vi "CD Init Outgoing Cyclic Signals.vi"(6 "Memory Table Offset":u32, 8 "error in":errorcluster, 9 "database":T1, 10 "can port":string, 11 "XNET Cluster":refnum<k21>) -> (0 "error out":errorcluster, 1 "Outgoing Cyclic Configuraiton":T5 {"Outgoing Cyclic Frame"."Transmit Propreties"."Transmit Time" format="%#_p"}, 2 "initial values":dbl[](array[numeric]), 3 "channels":refnum<class "TBM channel.lvclass">[](array[class]), 5 "outputs":T4[](array[typedef]), 7 "output IDs":string[](array[string]))   [LabVIEW 2013, in "J1939.lvlib"]
uses:
  J1939.lvlib
  CD Outgoing Cyclic Configuration.ctl
  CD Outgoing Cyclic Frame Pairs.ctl
  API Types/XNET Frame Event Properties.ctl
  module/configuration/Signal Mapping.ctl
  <vilib>/NI/Tag Bus/tag/Data Type.ctl
  <vilib>/NI/Tag Bus Module Framework/channel/TBM channel.lvclass
  CD Conversion Lookup Table Parameters Cluster.ctl
  Configuration/TypeDefs/J1939 db.ctl
  Configuration/TypeDefs/J1939 db frame.ctl
  Configuration/TypeDefs/J1939 db signal.ctl
  Configuration/TypeDefs/J1939 db frame direction.ctl
  <vilib>/NI/Tag Bus Module Framework/channel/channel classification.ctl
  <vilib>/NI/Tag Bus/tag/tag descriptor.lvclass/tag descriptor.ctl
  Frame Conversion/Common Conversions.vi
  Frame Conversion/Convert CAN Arb ID to J1939 ID.vi
  <vilib>/xnet/xnet.llb/XNET Create Session (Conversion).vi
  <resource>/objmgr/xnet.rc
  <vilib>/NI/Tag Bus/tag/tag descriptor.lvclass
  module/configuration/J1939 configuration.lvclass
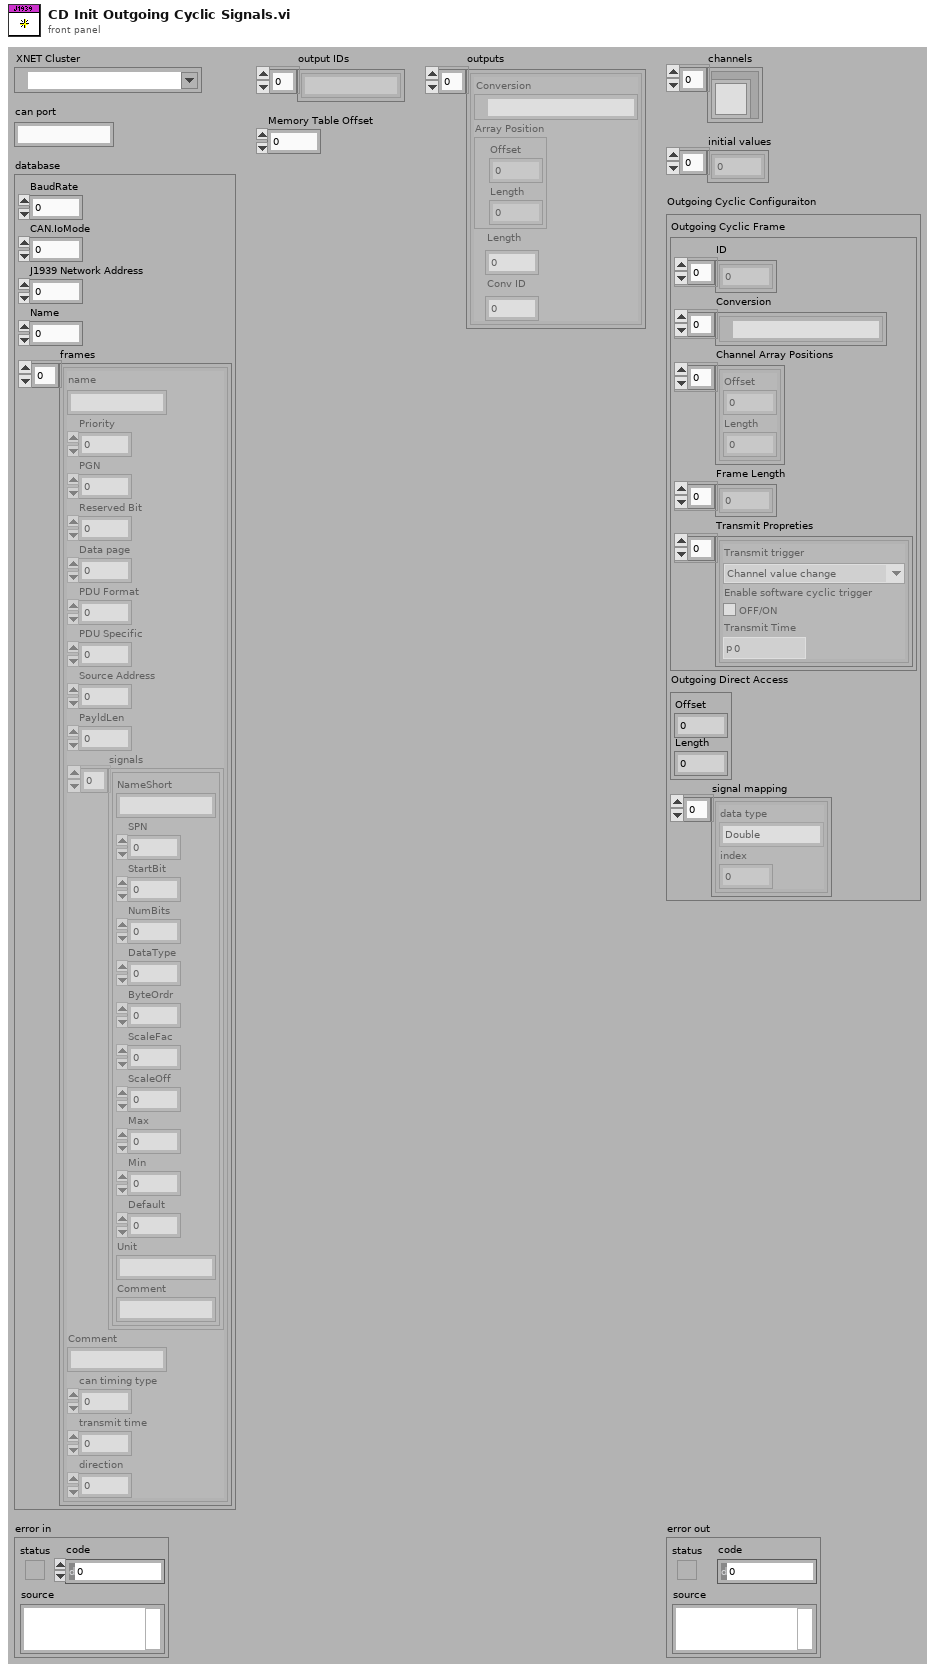
[diagram p1: front panel]
types:
  T1 = typedef "J1939.lvlib/J1939 db.ctl" = cluster{"BaudRate":u32, "CAN.IoMode":u32, "J1939 Network Address":u8, "Name":u64, "frames":T2[]}
  T2 = typedef "J1939.lvlib/J1939 db frame.ctl" = cluster{"name":string, "Priority":u8, "PGN":u32, "Reserved Bit":u8, "Data page":u8, "PDU Format":u8, "PDU Specific":u8, "Source Address":u8, "PayldLen":u32, "signals":T3[], "Comment":string, "can timing type":u32, "transmit time":dbl, "direction":u16}
  T3 = typedef "J1939.lvlib/J1939 db signal.ctl" = cluster{"NameShort":string, "SPN":i32, "StartBit":u32, "NumBits":u32, "DataType":u32, "ByteOrdr":u32, "ScaleFac":dbl, "ScaleOff":dbl, "Max":dbl, "Min":dbl, "Default":dbl, "Unit":string, "Comment":string}
  T4 = typedef "J1939.lvlib/CD Conversion Lookup Table Parameters Cluster.ctl" = cluster{"Conversion":refnum<k21>, "Array Position":cluster{"Offset":u32, "Length":u32}, "Length":u32, "Conv ID":u32}
  T5 = typedef "J1939.lvlib/CD Outgoing Cyclic Configuration.ctl" = cluster{"Outgoing Cyclic Frame":T6, "Outgoing Direct Access":cluster{"Offset":u32, "Length":u32}, "signal mapping":T8[]}
  T6 = typedef "J1939.lvlib/CD Outgoing Cyclic Frame Pairs.ctl" = cluster{"ID":u32[], "Conversion":refnum<k21>[], "Channel Array Positions":cluster{"Offset":u32, "Length":u32}[], "Frame Length":u32[], "Transmit Propreties":T7[]}
  T7 = typedef "J1939.lvlib/XNET Frame Event Properties.ctl" = cluster{"Transmit trigger":enum16{"Channel value change"}, "Enable software cyclic trigger":bool, "Transmit Time":dbl}
  T8 = typedef "J1939 configuration.lvclass/Signal Mapping.ctl" = cluster{"data type":T9, "index":i32}
  T9 = typedef "tag bus.lvlib/tag descriptor.lvclass/Data Type.ctl" = enum16{"Double", "Single", "I64", "I32", "I16", "I8", "U64", "U32", "U16", "U8", "Boolean", "String", "Array of Double", "Array of Single", "Array of I64", "Array of I32", "Array of I16", "Array of I8", "Array of U64", "Array of U32", "Array of U16", "Array of U8", "Array of Boolean", "Array of String"}
  T10 = typedef "J1939.lvlib/J1939 db frame direction.ctl" = enum16{"Input", "Output", "Input+Output"}
  T11 = typedef "TBM channel.lvclass/channel classification.ctl" = enum16{"input data", "output data", "processing parameter", "processing result"}
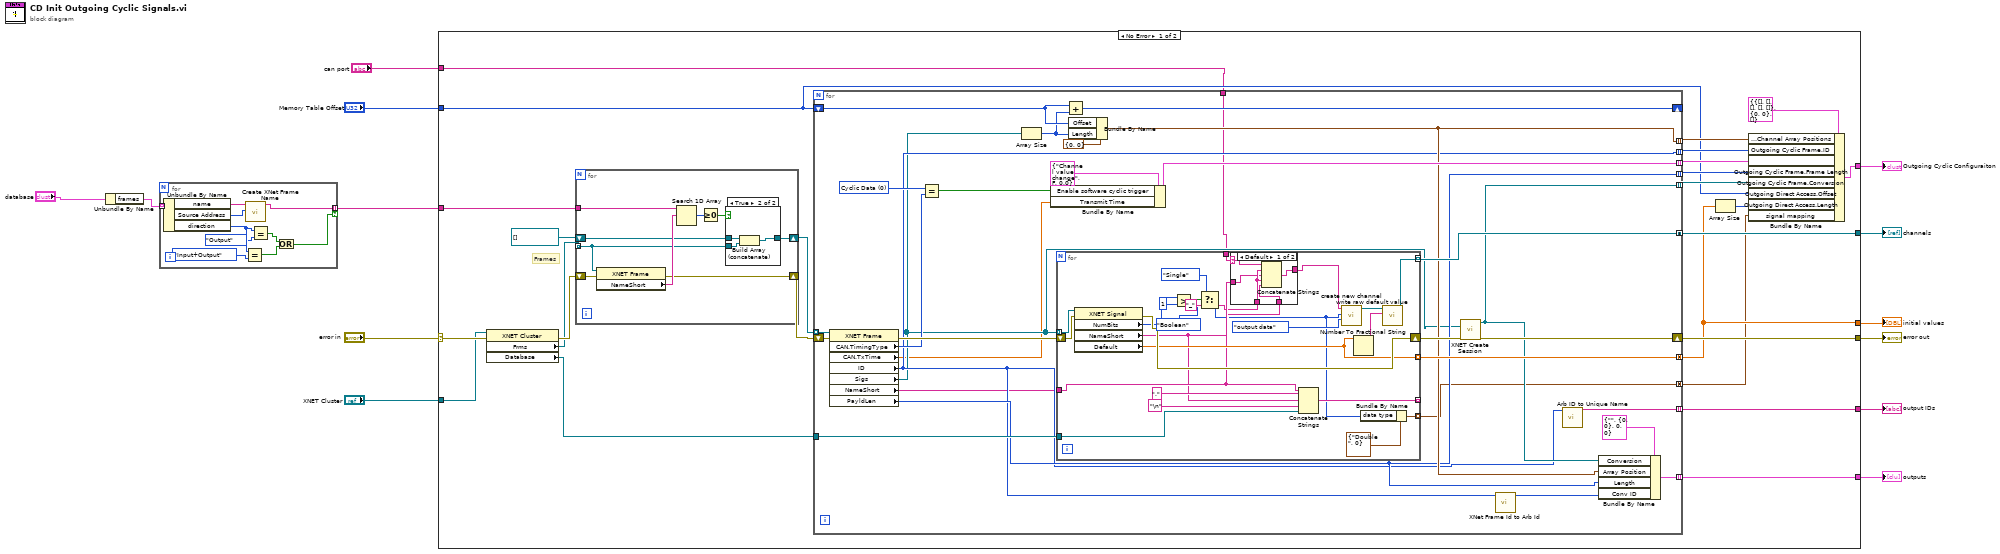
[diagram p0: block diagram]
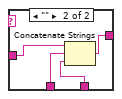
[diagram p3: hidden frame]
diagram:
  n1 = Unbundle By Name("database") -> ("frames"=w3:T2[])
  n2 = for {
    tunnel: w3 -> [w23] mode=indexing
    tunnel: [w20] -> w1 mode=indexing if=w14
    n3 = Unbundle By Name(w23) -> ("name"=w22:string, "Source Address"=w21:u8, "direction"=w19:u16)
    n4 = Equal?(x=w19, y=J1939_db_frame_direction."Input+Output" ("Direction")) -> (x = y?=w16:bool)
    n5 = call "Create XNet Frame Name.vi"("Source Address"=w21, "name"=w22) -> ("String"=w20:string)  [unwired: 8 in, 1 out]
    n6 = Equal?(x=w19, y=J1939_db_frame_direction."Output" ("Direction")) -> (x = y?=w15:bool)
    n7 = Or(x=w15, y=w16) -> (x .or. y?=w14:bool)
  }
  n8 = case shown="No Error" "error in" {
    selector: "error in" -> [w41 w126]
    tunnel: [w48 _] -> w11
    tunnel: [w39 w126] -> w13
    tunnel: "Memory Table Offset" -> [w30 _]
    tunnel: "XNET Cluster" -> [w40 _]
    tunnel: [w33 _] -> w9
    tunnel: [w32 _] -> w8
    tunnel: [w31 _] -> w7
    tunnel: [w29 _] -> w6
    tunnel: "can port" -> [w25 _]
    tunnel: w1 -> [w24 _]
    frame No Error {
      # "Frames"
      n9 = property class="XNET Cluster"(reference=w40, error in=w41) -> (error out=w38:errorcluster, "Frms"=w37:refnum<k21>[], "Database"=w26:refnum<k21>)  [unwired: 1 out]
      n10 = for {
        tunnel: w37 -> [w53] mode=indexing
        tunnel: w24 -> [w57]
        shift-right: [w52] -> w35
        shift-left: refnum<k21>[] [] -> [w49]
        shift-right: [w50] -> w34
        shift-left: w38 -> [w51]
        n11 = property class="XNET Frame"(reference=w53, error in=w51) -> (error out=w50:errorcluster, "NameShort"=w56:string)  [unwired: 1 out]
        n12 = Search 1D Array(1D array=w57, element=w56) -> (index of element=w55:i32)  [unwired: 1 in]
        n13 = Greater Or Equal To 0?(x=w55) -> (x >= 0?=w54:bool)
        n14 = case shown="True" w54 {
          tunnel: w49 -> [w58 w61]
          tunnel: w53 -> [_ w60]
          tunnel: [w58 w59] -> w52
          frame False {
          }
          frame True {
            n15 = Build Array (concatenate)(w61, w60) -> (w59:refnum<k21>[])
          }
        }
      }
      n16 = for {
        tunnel: [w73] -> w47 mode=indexing
        tunnel: [w69] -> w42 mode=indexing
        shift-right: [w91] -> _
        shift-left: w30 -> [w89]
        tunnel: [w72] -> w46 mode=indexing
        tunnel: [w71] -> w45 mode=indexing
        tunnel: [w79] -> w44 mode=indexing
        tunnel: w35 -> [w87] mode=indexing
        shift-right: [w82] -> w39
        shift-left: w34 -> [w86]
        tunnel: w26 -> [w81]
        tunnel: [w77] -> w33 mode=concatenating
        tunnel: [w76] -> w29 mode=concatenating
        tunnel: [w68] -> w32 mode=indexing
        tunnel: [w74] -> w31 mode=indexing
        tunnel: [w67] -> w27 mode=concatenating
        tunnel: w25 -> [w64]
        w83 = u32 0 items=["Cyclic Data", "Event Data", "Cyclic Remote", "Event Remote"] ("CAN:Timing Type")
        n17 = property class="XNET Frame"(reference=w87, error in=w86) -> (error out=w85:errorcluster, "CAN.TimingType"=w78:u32, "CAN.TxTime"=w62:dbl, "ID"=w69:u32, "Sigs"=w66:refnum<k21>[], "NameShort"=w65:string, "PayldLen"=w71:u32)  [unwired: 1 out]
        n18 = Equal?(x=w83, y=w78) -> (x = y?=w63:bool)
        n19 = Array Size(array=w66) -> (size(s)=w88:i32)
        n20 = Bundle By Name(cluster=T7 {"Transmit trigger"=enum."Channel value change", "Enable software cyclic trigger"=FALSE, "Transmit Time"=0.0} ("Cluster"), "Enable software cyclic trigger"=w63, "Transmit Time"=w62) -> (w79:T7)
        n21 = for {
          shift-right: [w113] -> w84
          shift-left: w85 -> [w114]
          tunnel: w66 -> [w115] mode=indexing
          tunnel: [w110] -> _ mode=indexing
          tunnel: w65 -> [w102]
          tunnel: [w106] -> w76 mode=indexing
          tunnel: w81 -> [w112]
          tunnel: [w109] -> w77 mode=indexing
          tunnel: [w104] -> w67 mode=indexing
          tunnel: w64 -> [w101]
          n22 = property class="XNET Signal"(reference=w115, error in=w114) -> (error out=w113:errorcluster, "NumBits"=w94:u32, "NameShort"=w98:string, "Default"=w106:dbl)  [unwired: 1 out]
          n23 = Greater?(x=w94, y=u32 1) -> (0:w97:bool)
          n24 = Select(t=Data_Type."Single" ("data type"), s=w97, f=Data_Type."Boolean" ("data type")) -> (s? t:f=w92:T9)
          n25 = case shown="Default" w101 {
            selector: w101 -> [w120 _]
            tunnel: w102 -> [w118 w125]
            tunnel: w98 -> [w117 w124]
            tunnel: "_" ("string") -> [w121 w123]
            tunnel: [w119 w122] -> w100
            frame Default {
              n26 = Concatenate Strings(w120, w121, w118, w121, w117) -> (w119:string)
            }
            frame "" {
              n27 = Concatenate Strings(w125, w123, w124) -> (w122:string)
            }
          }
          n28 = Concatenate Strings(w102, "." ("string"), w98, "\n" ("string"), w112) -> (w110:string)
          n29 = call <vilib>:"create new channel.vi"("channel classification"=channel_classification."output data", "data type"=w92, "channel name"=w100) -> ("channel"=w108:refnum<class "TBM channel.lvclass">)  [unwired: 8 in]
          n30 = Number To Fractional String(number=w106) -> (F-format string=w107:string)  [unwired: 3 in]
          n31 = Bundle By Name(cluster=T8 {"data type"=enum."Double", "index"=0}, "data type"=w92) -> (w104:T8)
          n32 = call <vilib>:"write raw default value.vi"("raw default"=w107, "system tag in"=w108) -> ("system tag out"=w109:refnum<class "TBM channel.lvclass">)  [unwired: 8 in, 1 out]
        }
        n33 = Add(x=w89, y=w88) -> (x+y=w91:u32)
        n34 = Bundle By Name(cluster=cluster{"Offset":u32, "Length":u32} {"Offset"=0, "Length"=0} ("Channel Array Position"), "Offset"=w89, "Length"=w88) -> (w72:cluster{"Offset":u32, "Length":u32})
        n35 = call-poly <vilib>:"XNET Create Session.vi"("signal list"=w66, "error in (no error)"=w84) -> ("session out"=w73:refnum<k21>, "error out"=w82:errorcluster)  [unwired: 12 in]
        n36 = call "XNet Frame Id to Arb Id.vi"("ID"=w69) -> ("Arb id"=w70:u32)  [unwired: 10 in]
        n37 = call "Arb ID to Unique Name.vi"("Arb ID"=w69) -> ("name"=w68:string)  [unwired: 10 in]
        n38 = Bundle By Name(cluster=T4 {"Conversion"="", "Array Position"={"Offset"=0, "Length"=0}, "Length"=0, "Conv ID"=0} ("Parameters"), "Conversion"=w73, "Array Position"=w72, "Length"=w71, "Conv ID"=w70) -> (w74:T4)
      }
      n39 = Array Size(array=w29) -> (size(s)=w28:i32)
      n40 = Bundle By Name(cluster=T5 {"Outgoing Cyclic Frame"={"ID"=[], "Conversion"=[], "Channel Array Positions"=[], "Frame Length"=[], "Transmit Propreties"=[]}, "Outgoing Direct Access"={"Offset"=0, "Length"=0}, "signal mapping"=[]} ("Outgoing Cyclic Configuraiton"), "Outgoing Cyclic Frame.Channel Array Positions"=w46, "Outgoing Cyclic Frame.ID"=w42, "Outgoing Cyclic Frame.Transmit Propreties"=w44, "Outgoing Cyclic Frame.Frame Length"=w45, "Outgoing Cyclic Frame.Conversion"=w47, "Outgoing Direct Access.Offset"=w30, "Outgoing Direct Access.Length"=w28, "signal mapping"=w27) -> (w48:T5)
    }
    frame Error {
    }
  }
  "error out" <- w13
  "Outgoing Cyclic Configuraiton" <- w11
  "channels" <- w9
  "output IDs" <- w8
  "outputs" <- w7
  "initial values" <- w6
